vi "Test Piccolo Raw Conversion.vi"() -> ()   [LabVIEW 2021, in "Piccolo.lvlib"]
uses:
  Piccolo.lvlib
panel:
  in  "Gate":u8
  out "Intensity Graph":u16[][](graph)
  in  "Pixel Y":u8 max=31
  in  "Pixel X":u8 max=31
  out "Waveform Graph":u16[](graph)
  out "Data":u16[][][](array[numeric])
  out "cancelled":bool
  out "Error Out":errorcluster
  in  "Error In":errorcluster
  in  "File Path":path
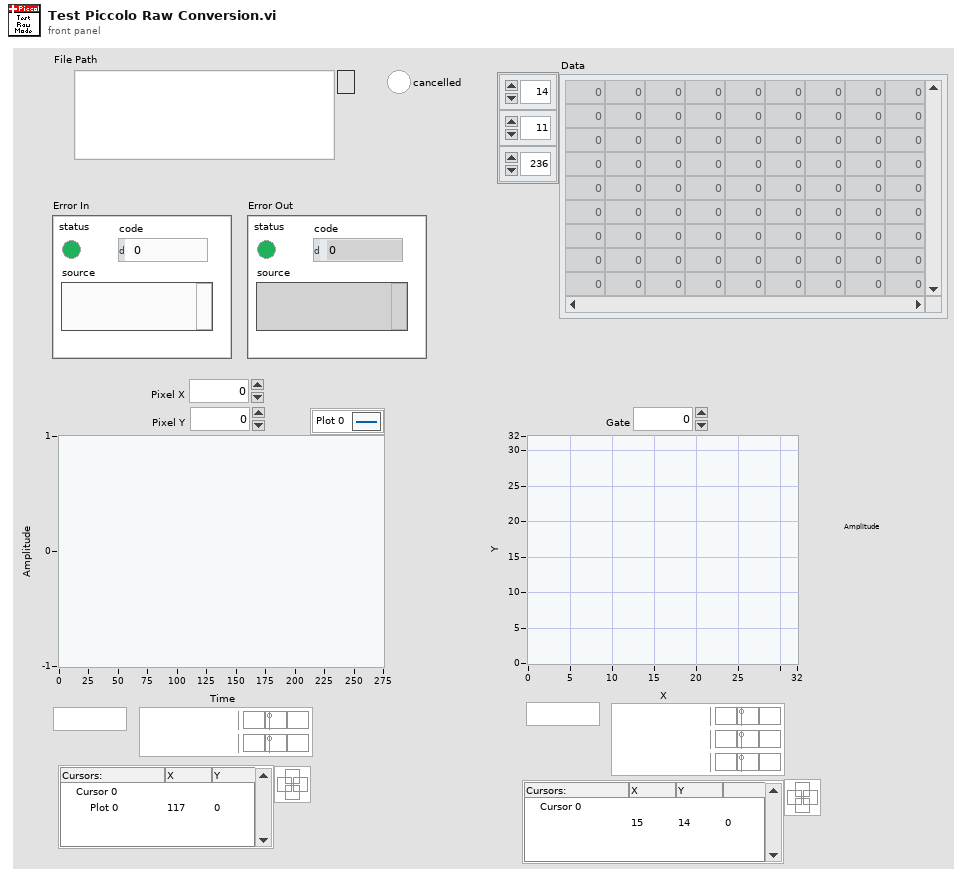
[diagram p1: front panel]
types:
  T1 = enum16{"big-endian, network order", "native, host order", "little-endian"}
  T2 = enum16{"open", "replace", "create", "open or create", "replace or create", "replace or create with confirmation"}
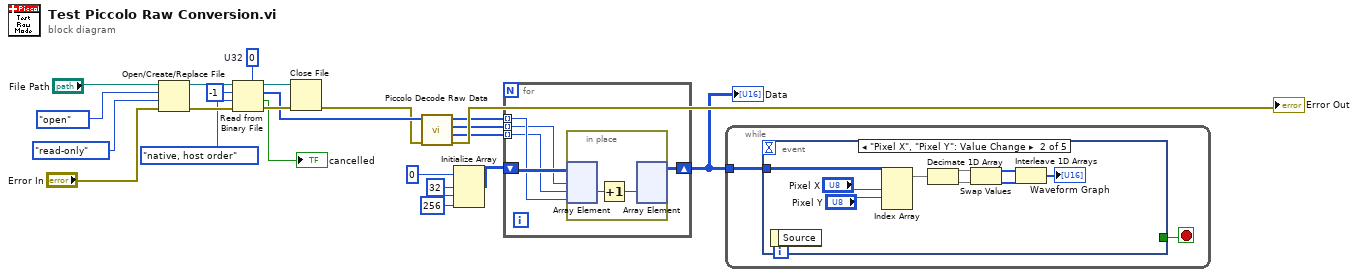
[diagram p0: block diagram]
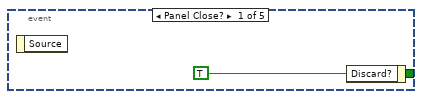
[diagram p2: hidden frame]
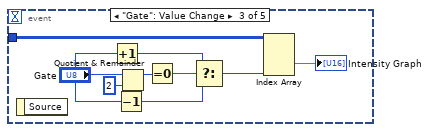
[diagram p3: hidden frame]
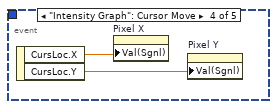
[diagram p4: hidden frame]
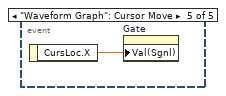
[diagram p5: hidden frame]
diagram:
  w7 = 32 ("dimension size")
  w17 = u32 0  # U32
  n1 = Open/Create/Replace File(file path (use dialog)="File Path", error in="Error In", operation (0:open)=T2."open", access (0:read/write)=enum16{"read/write", "read-only", "write-only"}."read-only") -> (refnum out=w19:refnum<file>, error out=w18:errorcluster)  [unwired: 2 in, 1 out]
  n2 = Read from Binary File(5:w17, 8:w18, 9:T1."native, host order" ("byte order (0:big-endian, network order)"), 10:-1 ("count (1)"), 11:w19) -> (0:w15:errorcluster, 1:→"cancelled":bool, 2:w12:u32[], 3:w16:refnum<file>)  [unwired: 1 in]
  n3 = Close File(refnum=w16, error in=w15) -> (error out=w11:errorcluster)  [unwired: 1 out]
  n4 = call "Piccolo Decode Raw Data.vi"("error in (no error)"=w11, "U32 Array"=w12) -> ("error out"=→"Error Out":errorcluster, "Y array"=w2:u8[], "X array"=w3:u8[], "TDC Bins"=w4:u16[])  [unwired: 5 in, 1 out]
  n5 = Initialize Array(u16 0 ("index"), w7, w7, 256 ("dimension size")) -> (w5:u16[][][])
  n6 = for {
    shift-right: [w24] -> w1
    shift-left: w5 -> [w28]
    tunnel: w4 -> [w27] mode=indexing
    tunnel: w3 -> [w26] mode=indexing
    tunnel: w2 -> [w25] mode=indexing
    n7 = in-place {
      n8 = in-place-array #1(w28, w26, w25, w27) -> (w30:u16)
      n9 = Increment(x=w30) -> (x+1=w29:u16)
      n10 = in-place-array #1(w29) -> (w24:u16[][][])  [unwired: 3 out]
    }
  }
  "Data" <- w1
  n11 = while {
    tunnel: w1 -> [w31]
    stop <- w32 stop-if-true
    n12 = event shown="[1] \"Pixel X\", \"Pixel Y\": Value Change" {
      selector: _ -> [_ _ _ _ _]
      dyn-events: _ -> [_ _ _ _ _]
      timeout: _ -> [_ _ _ _ _]
      tunnel: [w33 _ _ _ _] -> w32
      tunnel: w31 -> [_ w42 w51 _ _]
      event Panel Close? {
        w33 = TRUE ("Discard?")
        n13 = event-data() -> ()  [unwired: 1 in, 1 out]
        n14 = event-data("Discard?"=w33) -> ()  [unwired: 1 in, 1 out]
      }
      event "Pixel X", "Pixel Y": Value Change {
        n15 = event-data() -> ()  [unwired: 1 in, 1 out]
        n16 = Index Array(array=w42, index (dim 0)="Pixel X", index (dim 1)="Pixel Y") -> (element=w41:u16[])  [unwired: 1 in]
        n17 = Decimate 1D Array(w41) -> (w37:u16[], w36:u16[])
        n18 = Swap Values(12:w37, 14:w36) -> (1:w35:u16[], 3:w34:u16[])  [unwired: 1 in]
        n19 = Interleave 1D Arrays(w35, w34) -> (→"Waveform Graph":u16[])
      }
      event "Gate": Value Change {
        n20 = event-data() -> ()  [unwired: 1 in, 1 out]
        n21 = Increment(x="Gate") -> (x+1=w44:u8)
        n22 = Decrement(x="Gate") -> (x-1=w43:u8)
        n23 = Quotient & Remainder(x="Gate", y=u8 2) -> (x-y*floor(x/y)=w49:u8)  [unwired: 1 out]
        n24 = Equal To 0?(x=w49) -> (x = 0?=w48:bool)
        n25 = Select(t=w44, s=w48, f=w43) -> (s? t:f=w46:u8)
        n26 = Index Array(array=w51, index (dim 2)=w46) -> (element=→"Intensity Graph":u16[][])  [unwired: 2 in]
      }
      event "Intensity Graph": Cursor Move {
        n27 = event-data() -> ("CursLoc.X"=w53:dbl, "CursLoc.Y"=w52:dbl)  [unwired: 1 in]
        n28 = property on="Pixel X" class="DigNum (strict)"("Val(Sgnl)"=w53) -> ()  [unwired: 2 in, 2 out]
        n29 = property on="Pixel Y" class="DigNum (strict)"("Val(Sgnl)"=w52) -> ()  [unwired: 2 in, 2 out]
      }
      event "Waveform Graph": Cursor Move {
        n30 = event-data() -> ("CursLoc.X"=w54:dbl)  [unwired: 1 in]
        n31 = property on="Gate" class="DigNum (strict)"("Val(Sgnl)"=w54) -> ()  [unwired: 2 in, 2 out]
      }
    }
  }
